vi "Gunsim Precalc.vi"(2 "Robot Constants":T1={"Distance from Pivot Point to Drive Mount(in)"=2.0, "Distance from Pivot Point to Arm Mount(in)"=2.0, "Distance from Pivot Point to Launcher(in)"=2.0, "Distance from Pivot Point to Camera(in)"=2.0, "WheelEncoder Ticks/Revolution"=2.0, "Wheel Radius"=2.0, "Triangle Angle(degrees)"=2.0, "Minimum LA Distance(inches)"=2.0, "LA Distance/Tick(inches)"=2.0}, 3 "Framerate":i32, 4 "Other Constants":T3, 5 "Initial Velocity(in/s)":dbl) -> (0 "output cluster":T2, 1 "Wheel Power(ticks/100ms)":dbl)   [LabVIEW 2015]
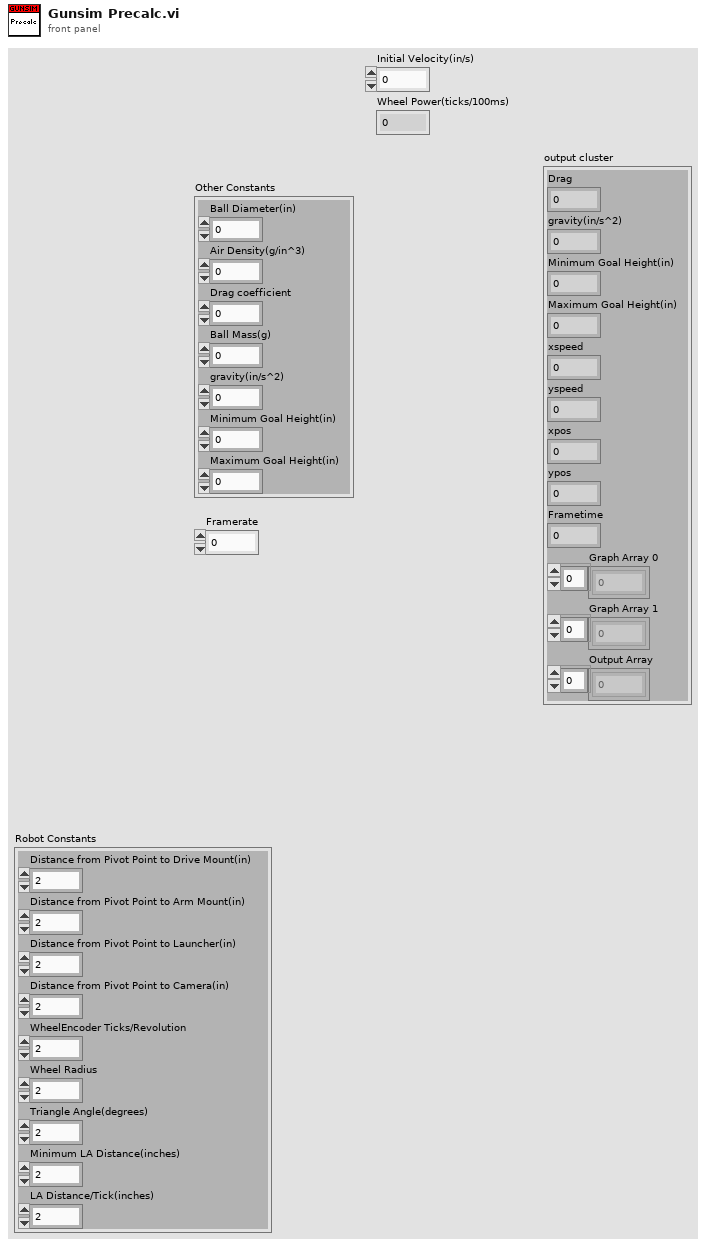
[diagram p1: front panel]
types:
  T1 = cluster{"Distance from Pivot Point to Drive Mount(in)":dbl, "Distance from Pivot Point to Arm Mount(in)":dbl, "Distance from Pivot Point to Launcher(in)":dbl, "Distance from Pivot Point to Camera(in)":dbl, "WheelEncoder Ticks/Revolution":dbl, "Wheel Radius":dbl, "Triangle Angle(degrees)":dbl, "Minimum LA Distance(inches)":dbl, "LA Distance/Tick(inches)":dbl}
  T2 = cluster{"Drag":dbl, "gravity(in/s^2)":dbl, "Minimum Goal Height(in)":dbl, "Maximum Goal Height(in)":dbl, "xspeed":dbl, "yspeed":dbl, "xpos":dbl, "ypos":dbl, "Frametime":dbl, "Graph Array 0":dbl[], "Graph Array 1":dbl[], "Output Array":dbl[]}
  T3 = cluster{"Ball Diameter(in)":dbl, "Air Density(g/in^3)":dbl, "Drag coefficient":dbl, "Ball Mass(g)":dbl, "gravity(in/s^2)":dbl, "Minimum Goal Height(in)":dbl, "Maximum Goal Height(in)":dbl}
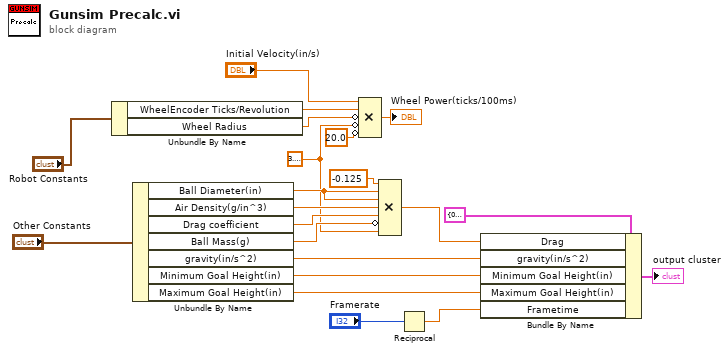
[diagram p0: block diagram]
diagram:
  w5 = 3.141592653589793
  n1 = Unbundle By Name("Robot Constants") -> ("WheelEncoder Ticks/Revolution"=w4:dbl, "Wheel Radius"=w3:dbl)
  n2 = Unbundle By Name("Other Constants") -> ("Ball Diameter(in)"=w11:dbl, "Air Density(g/in^3)"=w12:dbl, "Drag coefficient"=w13:dbl, "Ball Mass(g)"=w14:dbl, "gravity(in/s^2)"=w17:dbl, "Minimum Goal Height(in)"=w18:dbl, "Maximum Goal Height(in)"=w19:dbl)
  n3 = Compound Arithmetic op=MULTIPLY("Initial Velocity(in/s)", w4, invert w3, invert w5, invert 20.0 ("value")) -> (→"Wheel Power(ticks/100ms)":dbl)
  n4 = Compound Arithmetic op=MULTIPLY(-0.125 ("value"), w11, w11, w12, w13, invert w14, w5) -> (w15:dbl)
  n5 = Reciprocal(x="Framerate") -> (1/x=w21:dbl)
  n6 = Bundle By Name(cluster=T2 {"Drag"=0.0, "gravity(in/s^2)"=-386.09, "Minimum Goal Height(in)"=85.0, "Maximum Goal Height(in)"=109.0, "xspeed"=0.0, "yspeed"=0.0, "xpos"=0.0, "ypos"=0.0, "Frametime"=0.0, "Graph Array 0"=[], "Graph Array 1"=[], "Output Array"=[]}, "Drag"=w15, "gravity(in/s^2)"=w17, "Minimum Goal Height(in)"=w18, "Maximum Goal Height(in)"=w19, "Frametime"=w21) -> (→"output cluster":T2)
